vi "Configure Bus Source (RS232).vi"(0 "VISA resource name":refnum<visa-resource-name>, 1 "Polarity (0: Normal)":u16(ring) items=["Normal", "Inverted"], 2 "Parity (0: None)":u16(ring) items=["None", "Even", "Odd"], 3 "Custom Bit Rate (9600 bps)":dbl=9600.0, 5 "BUS Number (9: Bus 1)":u16(ring)=9 items=["Bus 1"=9, "Bus 2"=10, "Bus 3"=11, "Bus 4"=12], 7 "RX Source (0: Channel 1)":u16(ring) items=["Channel 1"=0, "Channel 2"=1, "Channel 3"=2, "Channel 4"=3, "Digital Channel 0"=14, "Digital Channel 1"=15, "Digital Channel 2"=16, "Digital Channel 3"=17, "Digital Channel 4"=18, "Digital Channel 5"=19, "Digital Channel 6"=20, "Digital Channel 7"=21, "Digital Channel 8"=22, "Digital Channel 9"=23, "Digital Channel 10"=24, "Digital Channel 11"=25, "Digital Channel 12"=26, "Digital Channel 13"=27, "Digital Channel 14"=28, "Digital Channel 15"=29, "Off"=30], 9 "TX Source (1: Channel 2)":u16(ring)=1 items=["Channel 1"=0, "Channel 2"=1, "Channel 3"=2, "Channel 4"=3, "Digital Channel 0"=14, "Digital Channel 1"=15, "Digital Channel 2"=16, "Digital Channel 3"=17, "Digital Channel 4"=18, "Digital Channel 5"=19, "Digital Channel 6"=20, "Digital Channel 7"=21, "Digital Channel 8"=22, "Digital Channel 9"=23, "Digital Channel 10"=24, "Digital Channel 11"=25, "Digital Channel 12"=26, "Digital Channel 13"=27, "Digital Channel 14"=28, "Digital Channel 15"=29, "Off"=30], 11 "error in (no error)":errorcluster, 12 "Data Bits (0: 7 Bits)":u16(ring) items=["7 Bits", "8 Bits", "9 Bits"], 13 "Delimiter (5: Off)":u16(ring)=5 items=["0x00 (Null)", "0x0A (LF)", "0x0D (CR)", "0xFF (XFF)", "0x20 (Space)", "Off"], 14 "Bit Rate (0:2765.8 Kbps)":u16(ring) items=["2765.8 Kbps", "1843.2 Kbps", "1382.4 Kbps", "921.6 Kbps", "460.8 Kbps", "230.4 Kbps", "128 Kbps", "115.2 Kbps", "57.6 Kbps", "56 Kbps", "38.4 Kbps", "28.8 Kbps", "19.2 Kbps", "15.2 Kbps", "14.4 Kbps", "9.6 Kbps", "7.2 Kbps", "4.8 Kbps", "3.6 Kbps", "2.4 Kbps", "2 Kbps", "1.8 Kbps", "1.2 Kbps", "600 bps", "300 bps", "150 bps", "134 bps", "110 bps", "75 bps", "50 bps", "Custom"]) -> (4 "VISA resource name out":refnum<visa-resource-name>, 15 "error out":errorcluster)   [LabVIEW 2009, in "Tektronix DPO MSO 2000 4000 Series.lvlib"]
doc: "Configures RS232 bus settings for an oscilloscope."
uses:
  <instrlib>/Tektronix DPO MSO 2000 4000 Series/Tektronix DPO MSO 2000 4000 Series.lvlib
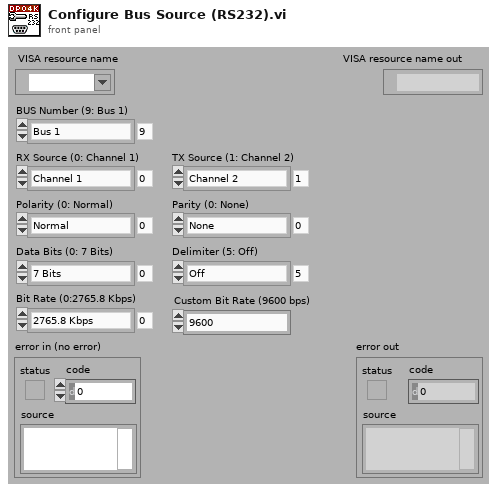
[diagram p1: front panel]
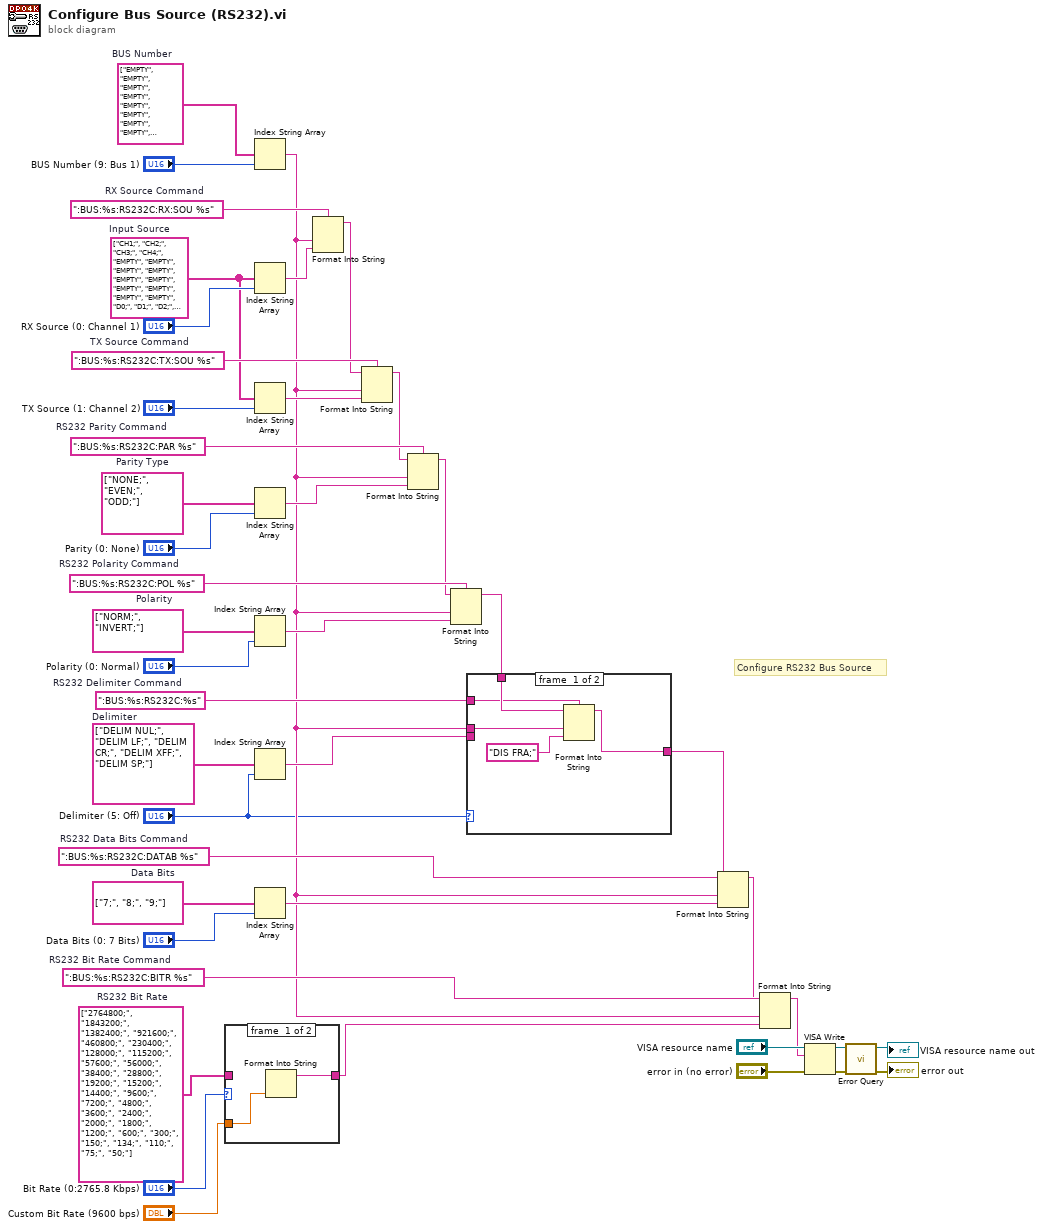
[diagram p0: block diagram]
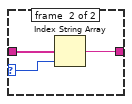
[diagram p2: hidden frame]
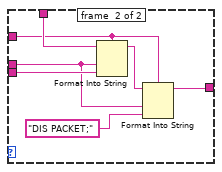
[diagram p3: hidden frame]
diagram:
  w10 = ":BUS:%s:RS232C:DATAB %s"  # RS232 Data Bits Command
  w12 = string[] ["7;", "8;", "9;"]  # Data Bits
  w13 = ":BUS:%s:RS232C:%s"  # RS232 Delimiter Command
  w14 = string[] ["DELIM NUL;", "DELIM LF;", "DELIM CR;", "DELIM XFF;", "DELIM SP;"]  # Delimiter
  w21 = ":BUS:%s:RS232C:POL %s"  # RS232 Polarity Command
  w22 = string[] ["NONE;", "EVEN;", "ODD;"]  # Parity Type
  w31 = ":BUS:%s:RS232C:TX:SOU %s"  # TX Source Command
  w32 = string[] ["EMPTY", "EMPTY", "EMPTY", "EMPTY", "EMPTY", "EMPTY", "EMPTY", "EMPTY", "EMPTY", "B1", "B2", "B3", "B4"]  # BUS Number
  w20 = string[] ["NORM;", "INVERT;"]  # Polarity
  w42 = ":BUS:%s:RS232C:PAR %s"  # RS232 Parity Command
  w41 = ":BUS:%s:RS232C:BITR %s"  # RS232 Bit Rate Command
  w43 = ":BUS:%s:RS232C:RX:SOU %s"  # RX Source Command
  w28 = string[] ["CH1;", "CH2;", "CH3;", "CH4;", "EMPTY", "EMPTY", "EMPTY", "EMPTY", "EMPTY", "EMPTY", "EMPTY", "EMPTY", "EMPTY", "EMPTY", "D0;", "D1;", "D2;", "D3;", "D4;", "D5;", "D6;", "D7;", "D8;", "D9;", "D10;", "D11;", "D12;", "D13;", "D14;", "D15;", "OFF;"]  # Input Source
  w34 = string[] ["2764800;", "1843200;", "1382400;", "921600;", "460800;", "230400;", "128000;", "115200;", "57600;", "56000;", "38400;", "28800;", "19200;", "15200;", "14400;", "9600;", "7200;", "4800;", "3600;", "2400;", "2000;", "1800;", "1200;", "600;", "300;", "150;", "134;", "110;", "75;", "50;"]  # RS232 Bit Rate
  # "Configure RS232 Bus Source"
  n1 = case shown="0..29, Default" "Bit Rate (0:2765.8 Kbps)" {
    selector: "Bit Rate (0:2765.8 Kbps)" -> [_ w47]
    tunnel: w34 -> [_ w49]
    tunnel: [w46 w48] -> w5
    tunnel: "Custom Bit Rate (9600 bps)" -> [w45 _]
    frame #0 {
      n2 = Format Into String(w45) -> (resulting string=w46:string)  [unwired: 3 in, 1 out]
    }
    frame #1 {
      n3 = Index String Array(1:w47, 2:w49) -> (0:w48:string)  [unwired: 1 in]
    }
  }
  n4 = Index String Array(1:"BUS Number (9: Bus 1)", 2:w32) -> (0:w8:string)  [unwired: 1 in]
  n5 = Index String Array(1:"RX Source (0: Channel 1)", 2:w28) -> (0:w27:string)  [unwired: 1 in]
  n6 = Index String Array(1:"TX Source (1: Channel 2)", 2:w28) -> (0:w25:string)  [unwired: 1 in]
  n7 = Index String Array(1:"Parity (0: None)", 2:w22) -> (0:w24:string)  [unwired: 1 in]
  n8 = Index String Array(1:"Polarity (0: Normal)", 2:w20) -> (0:w18:string)  [unwired: 1 in]
  n9 = Index String Array(1:"Delimiter (5: Off)", 2:w14) -> (0:w16:string)  [unwired: 1 in]
  n10 = Index String Array(1:"Data Bits (0: 7 Bits)", 2:w12) -> (0:w9:string)  [unwired: 1 in]
  n11 = Format Into String(format string=w43, w8, w27) -> (resulting string=w26:string)  [unwired: 2 in, 1 out]
  n12 = Format Into String(format string=w31, initial string=w26, w8, w25) -> (resulting string=w23:string)  [unwired: 1 in, 1 out]
  n13 = Format Into String(format string=w42, initial string=w23, w8, w24) -> (resulting string=w17:string)  [unwired: 1 in, 1 out]
  n14 = Format Into String(format string=w21, initial string=w17, w8, w18) -> (resulting string=w15:string)  [unwired: 1 in, 1 out]
  n15 = case shown="0..4" "Delimiter (5: Off)" {
    tunnel: w16 -> [_ w61]
    tunnel: w15 -> [w54 w60]
    tunnel: w13 -> [w52 w58]
    tunnel: w8 -> [w51 w57]
    tunnel: [w53 w55] -> w7
    frame #0 {
      n16 = Format Into String(format string=w52, initial string=w54, w51, "DIS FRA;" ("input 2")) -> (resulting string=w53:string)  [unwired: 1 in, 1 out]
    }
    frame #1 {
      n17 = Format Into String(format string=w58, initial string=w60, w57, w61) -> (resulting string=w59:string)  [unwired: 1 in, 1 out]
      n18 = Format Into String(format string=w58, initial string=w59, w57, "DIS PACKET;" ("input 2")) -> (resulting string=w55:string)  [unwired: 1 in, 1 out]
    }
  }
  n19 = Format Into String(format string=w10, initial string=w7, w8, w9) -> (resulting string=w6:string)  [unwired: 1 in, 1 out]
  n20 = Format Into String(format string=w41, initial string=w6, w8, w5) -> (resulting string=w4:string)  [unwired: 1 in, 1 out]
  n21 = VISA Write(VISA resource name="VISA resource name", write buffer=w4, error in (no error)="error in (no error)") -> (VISA resource name out=w40:refnum<visa-resource-name>, error out=w39:errorcluster)  [unwired: 1 out]
  n22 = call <instrlib>:"Error Query.vi"("error in (no error)"=w39, "VISA resource name"=w40) -> ("error out"=→"error out":errorcluster, "VISA resource name out"=→"VISA resource name out":refnum<visa-resource-name>)  [unwired: 6 in, 2 out]
